vi "Init 2D Array.vi"(6 "Length":i32, 7 "1D Array Element":i32[](array[numeric])) -> (1 "2D Array":i32[][](array[numeric]))   [LabVIEW 2019]
doc: "Given a 1D Array, initialize a 2D array of Length elements of 1D Array (e.g. given 1D array [1,2,3] and length=2... [[1,2,3], [1,2,3]])."
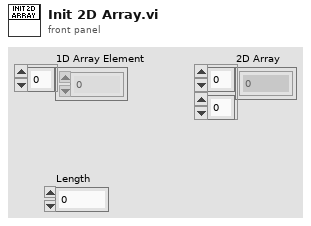
[diagram p1: front panel]
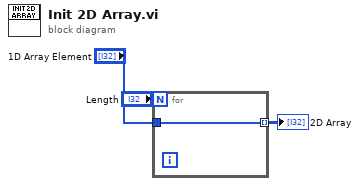
[diagram p0: block diagram]
diagram:
  n1 = for {
    N: "Length" -> [_]
    tunnel: "1D Array Element" -> [w4]
    tunnel: [w4] -> w3 mode=indexing
  }
  "2D Array" <- w3
